vi "test Get and Set Allow Echo Frames.vi"(11 "Test Case In":refnum<class "Test PCANBasic.lvclass">) -> (0 "error out":errorcluster, 3 "Test Case Out":refnum<class "Test PCANBasic.lvclass">)   [LabVIEW 2020, in "Test PCANBasic.lvclass"]
uses:
  <vilib>/Astemes/LUnit/Test Case.lvclass/Test Case.ctl
  Test PCANBasic.lvclass
  Test PCANBasic.lvclass/Test PCANBasic.ctl
  C:/Program Files/National Instruments/LabVIEW 2026/vi.lib/Astemes/LUnit/Test Case.lvclass
  C:/Program Files/National Instruments/LabVIEW 2026/vi.lib/Astemes/LUnit/LUnit Runnable.lvclass
  D:/git/PCAN-Basic-LabVIEW/tests/Tests PCANBasic/Test PCANBasic.lvclass
  source/PCANBasic.lvlib
  Global PCAN Channel.vi
  Global PCAN Baudrate.vi
  <vilib>/Astemes/LUnit/Test Case.lvclass
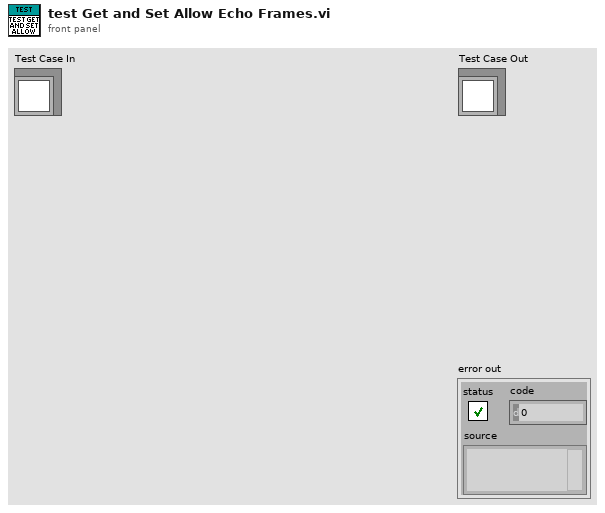
[diagram p1: front panel]
types:
  T1 = typedef "PCANBasic.lvlib/PCAN Baud.ctl" = u16
  T2 = typedef "PCANBasic.lvlib/TPCANHandle.ctl" = u16
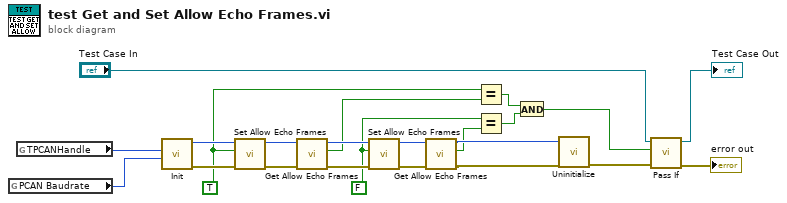
[diagram p0: block diagram]
diagram:
  w6 = FALSE ("Enable")
  w4 = TRUE ("Enable")
  n1 = global read "Global PCAN Baudrate.vi" "PCAN Baudrate"() -> (w20:T1)
  n2 = global read "Global PCAN Channel.vi" "TPCANHandle"() -> (w19:T2)
  n3 = call "Init.vi"("Baudrate"=w20, "Channel"=w19) -> ("error out"=w18:errorcluster, "TPCANHandle out"=w16:T2)  [unwired: 7 in, 1 out]
  n4 = call "Set Allow Echo Frames.vi"("error in"=w18, "Enable"=w4, "TPCANHandle in"=w16) -> ("error out"=w17:errorcluster, "TPCANHandle out"=w14:T2)  [unwired: 6 in, 1 out]
  n5 = call "Get Allow Echo Frames.vi"("error in"=w17, "TPCANHandle in"=w14) -> ("error out"=w15:errorcluster, "Enabled"=w5:bool, "TPCANHandle out"=w11:T2)  [unwired: 6 in, 1 out]
  n6 = call "Set Allow Echo Frames.vi"("error in"=w15, "Enable"=w6, "TPCANHandle in"=w11) -> ("error out"=w12:errorcluster, "TPCANHandle out"=w10:T2)  [unwired: 6 in, 1 out]
  n7 = call "Get Allow Echo Frames.vi"("error in"=w12, "TPCANHandle in"=w10) -> ("error out"=w9:errorcluster, "Enabled"=w7:bool, "TPCANHandle out"=w8:T2)  [unwired: 6 in, 1 out]
  n8 = Equal?(x=w4, y=w5) -> (x = y?=w2:bool)
  n9 = Equal?(x=w6, y=w7) -> (x = y?=w3:bool)
  n10 = And(x=w2, y=w3) -> (x .and. y?=w1:bool)
  n11 = call "Uninitialize.vi"("error in"=w9, "TPCANHandle in"=w8) -> ("error out"=w13:errorcluster)  [unwired: 8 in, 1 out]
  n12 = call <vilib>:"Pass If.vi"("error in (no error)"=w13, "Pass?"=w1, "LUnit Test Case In"="Test Case In") -> ("error out"=→"error out":errorcluster, "LUnit Test Case Out"=→"Test Case Out":refnum<class "Test PCANBasic.lvclass">)  [unwired: 7 in]
